vi "DDS Output Enable.vi"(10 "enable":i32, 11 "channel_index":u8) -> ()   [LabVIEW 2021, in "vmmso.lvlib"]
doc: "DLL_API void WINAPI DDSOutputEnable(unsigned char channel_index, int enable);"
uses:
  vmmso.lvlib
  vmmso.dll
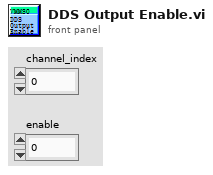
[diagram p1: front panel]
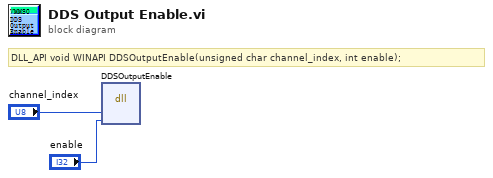
[diagram p0: block diagram]
diagram:
  # "DLL_API void WINAPI DDSOutputEnable(unsigned char channel_index, int enable);"
  n1 = dll-call lib="D:/labviewdemo/LabviewDemo 21/vmmso/vmmso.*" fn="DDSOutputEnable"("channel_index"="channel_index", "enable"="enable") -> ()  [unwired: 6 in, 2 out]
